vi "MoveTime.vi"(5 "DC Motor 2":T2, 7 "DC Motor":T2, 8 "Time (ms)":u32, 9 "Pwr Blue":i8, 10 "Pwr Red":i8, 11 "NXT In":T3) -> (3 "NXT Out":T3={"Hardware"="NXT", "Flattened String"=""})   [LabVIEW 2010]
uses:
  <vilib>/NXT/Subs/LVHSConnector.ctl
  <vilib>/NXT/Subs/MotorXNode.DC Motor Type.ctl
  <vilib>/NXT/NXTIO Xnodes/NXTIOXNode/NXTIO.xnode
  <vilib>/NXT/Subs/MotorXNode.2DCMotor.ctl
  <vilib>/NXT/NXTIO Xnodes/NXTIONodeSubVIs/TETRIX IO Move DC Motors.vi
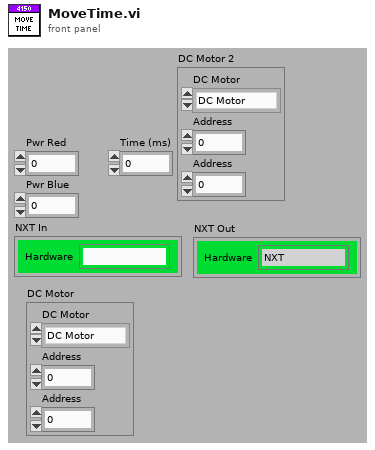
[diagram p1: front panel]
types:
  T1 = typedef "MotorXNode.DC Motor Type.ctl" = enum16{"DC Motor"}
  T2 = cluster{"DC Motor":T1, "Address":i16, "Address":i16}
  T3 = typedef "LVHSConnector.ctl" = cluster{"Hardware":string, "Flattened String":string}
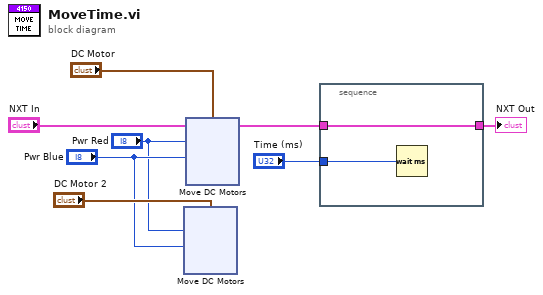
[diagram p0: block diagram]
diagram:
  n1 = xnode "Move DC Motors"("Power/Speed 2"="Pwr Blue", "Power/Speed 1"="Pwr Red", "Motors"="DC Motor 2") -> ()  [unwired: 1 in, 1 out]
  n2 = xnode "Move DC Motors"("Power/Speed 2"="Pwr Blue", "Power/Speed 1"="Pwr Red", "Motors"="DC Motor", "NXT"="NXT In") -> ("NXT"=w7:T3)
  n3 = stacked-sequence {
    tunnel: w7 -> [w10]
    tunnel: [w10] -> w6
    tunnel: "Time (ms)" -> [w9]
    frame #0 {
      n4 = Wait (ms)(milliseconds to wait=w9) -> ()  [unwired: 1 out]
    }
  }
  "NXT Out" <- w6
